vi "Check VI Version.vi"(0 "LabVIEW version":string, 5 "VI path":path, 11 "error in (no error)":errorcluster) -> (4 "Incompatible version warning":string, 15 "error out":errorcluster)   [LabVIEW 2021, in "Converter.lvlib"]
uses:
  Converter.lvlib
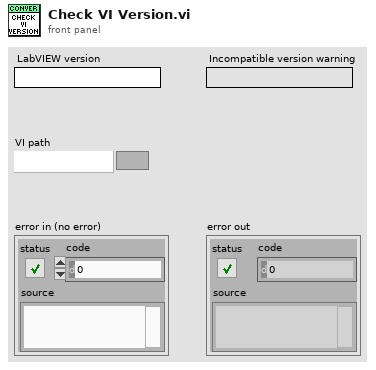
[diagram p1: front panel]
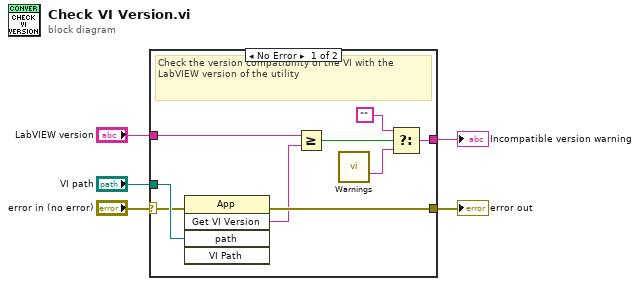
[diagram p0: block diagram]
diagram:
  n1 = case shown="No Error" "error in (no error)" {
    selector: "error in (no error)" -> [w6 w15]
    tunnel: [w14 w15] -> w5
    tunnel: [w13 _] -> w4
    tunnel: "LabVIEW version" -> [w9 _]
    tunnel: "VI path" -> [w7 _]
    frame No Error {
      # "Check the version compatibility of the VI with the LabVIEW version of the utility"
      n2 = invoke class="App" method="Get VI Version"(error in=w6, "path"=w7) -> (error out=w14:errorcluster, "GetVIVers"=w8:string)  [unwired: 3 in, 3 out]
      n3 = Greater Or Equal?(x=w9, y=w8) -> (x >= y?=w10:bool)
      n4 = call "Warnings.vi"() -> ("Incompatible measurement version"=w12:string)  [unwired: 8 in, 7 out]
      n5 = Select(t="", s=w10, f=w12) -> (s? t:f=w13:string)
    }
    frame Error {
      # "Pass"
    }
  }
  "error out" <- w5
  "Incompatible version warning" <- w4
